vi "trusted client certfications.vi"(8 "Error In":errorcluster, 10 "OPC UA server refnum in":refnum<k21>, 11 "DOM document in":refnum<k20>) -> (0 "Error Out":errorcluster, 1 "trusted client certfications":path[](array[path]), 2 "OPC UA server refnum out":refnum<k21>, 3 "DOM document out":refnum<k20>)   [LabVIEW 2013, in "OPCUA XML.lvlib"]
uses:
  OPCUA XML.lvlib
  <vilib>/xml/Close Reference(Node).vi
  <resource>/objmgr/DOMUserDefRef.rc
  <vilib>/xml/NI_XML.lvlib
  <vilib>/OPCUA/NI OPC UA Server.lvlib
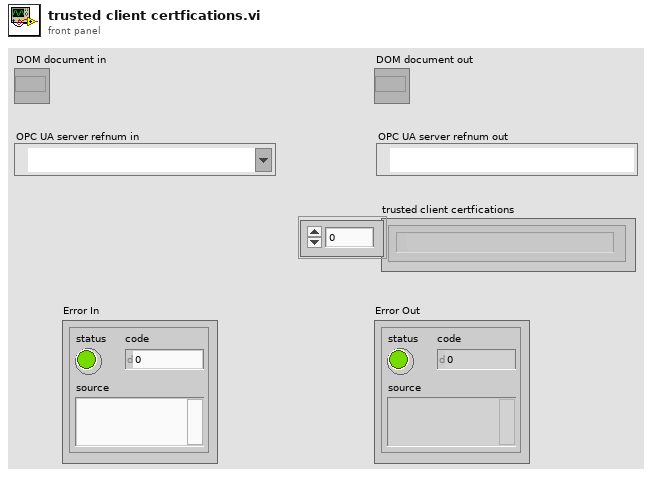
[diagram p1: front panel]
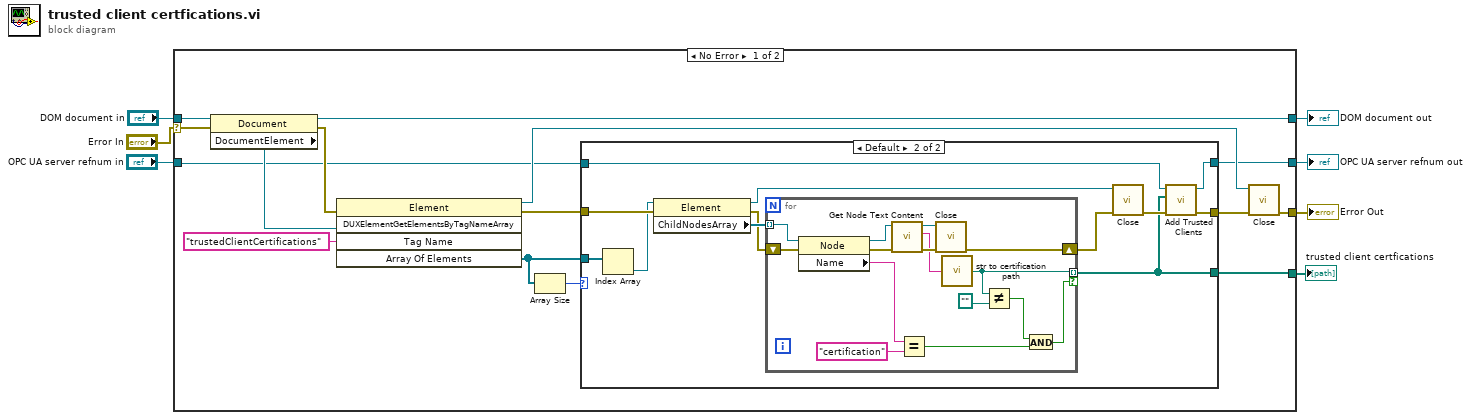
[diagram p0: block diagram]
diagram:
  n1 = case shown="No Error" "Error In" {
    selector: "Error In" -> [w22 w54]
    tunnel: [w19 w54] -> w7
    tunnel: "DOM document in" -> [w21 w53]
    tunnel: [w20 w53] -> w4
    tunnel: [w10 w52] -> w3
    tunnel: "OPC UA server refnum in" -> [w9 w52]
    tunnel: [w8 _] -> w1
    frame No Error {
      n2 = property class="Document"(reference=w21, error in=w22) -> (reference out=w20:refnum<k20>, error out=w14:errorcluster, "DocumentElement"=w16:refnum<k20>)
      n3 = invoke class="Element" method="DUXElementGetElementsByTagNameArray"(reference=w16, error in=w14, "Tag Name"="trustedClientCertifications") -> (reference out=w13:refnum<k20>, error out=w17:errorcluster, "Array Of Elements"=w12:refnum<k20>[])  [unwired: 2 in, 2 out]
      n4 = Array Size(array=w12) -> (size(s)=w11:i32)
      n5 = case shown="Default" w11 {
        tunnel: [w24 w28] -> w18
        tunnel: w17 -> [w24 w36]
        tunnel: w12 -> [_ w31]
        tunnel: [w23 w27] -> w10
        tunnel: w9 -> [w23 w26]
        tunnel: [_ w25] -> w8
        frame 0 {
        }
        frame Default {
          n6 = Index Array(array=w31) -> (element=w30:refnum<k20>)  [unwired: 1 in]
          n7 = property class="Element"(reference=w30, error in=w36) -> (reference out=w35:refnum<k20>, error out=w33:errorcluster, "ChildNodesArray"=w34:refnum<k20>[])
          n8 = for {
            tunnel: w34 -> [w48] mode=indexing
            tunnel: [w40] -> w25 mode=indexing if=w38
            shift-right: [w49] -> w32
            shift-left: w33 -> [w47]
            n9 = property class="Node"(reference=w48, error in=w47) -> (reference out=w46:refnum<k20>, error out=w42:errorcluster, "Name"=w45:string)
            n10 = call <vilib>:"Get Node Text Content.vi"("error in (no error)"=w42, "node in"=w46) -> ("error out"=w51:errorcluster, "node text"=w41:string, "node out"=w50:refnum<k20>)  [unwired: 7 out]
            n11 = Equal?(x=w45, y="certification") -> (x = y?=w43:bool)
            n12 = call-poly <vilib>:"Close.vi"("error in (no error)"=w51, "node"=w50) -> ("error out"=w49:errorcluster)  [unwired: 7 out]
            n13 = call "str to certification path.vi"("node text"=w41) -> ("File Path Control"=w40:path)  [unwired: 4 in]
            n14 = Not Equal?(x=w40, y=path "") -> (x != y?=w37:bool)
            n15 = And(x=w37, y=w43) -> (x .and. y?=w38:bool)
          }
          n16 = call-poly <vilib>:"Close.vi"("error in (no error)"=w32, "node"=w35) -> ("error out"=w29:errorcluster)  [unwired: 7 out]
          n17 = call <vilib>:"Add Trusted Clients.vi"("error in (no error)"=w29, "trusted client certificates"=w25, "OPC UA server refnum in"=w26) -> ("error out"=w28:errorcluster, "OPC UA server refnum out"=w27:refnum<k21>)  [unwired: 7 in]
        }
      }
      n18 = call-poly <vilib>:"Close.vi"("error in (no error)"=w18, "node"=w13) -> ("error out"=w19:errorcluster)  [unwired: 7 out]
    }
    frame Error {
    }
  }
  "Error Out" <- w7
  "DOM document out" <- w4
  "OPC UA server refnum out" <- w3
  "trusted client certfications" <- w1
